vi "Convert Dirs to VI Libraries (proxy)__ogtk.vi"(8 "error in (no error)":errorcluster, 11 "directories":path[](array[path])) -> (0 "error out":errorcluster)   [LabVIEW 2011]
doc: "Converts an array of Directories into VI Library (.llb) files. \n\nNote: This VI dynamically calls the LabVIEW subVI \"Convert Dirs to VI Libraries.vi\" located at <LabVIEW>\\project\\llbedit.llb (as it is not in the VI search paths)."
uses:
  Convert File Extension (Path)__ogtk.vi
panel:
  in  "type specifier":refnum<vi>
  # "Convert Dirs to VI Libraries (proxy).vi\n\nCalls \"Convert Dirs to VI Libraries.vi\" by reference\n\nPlease visit http://www.OpenG.org to learn about the\nOpen Source LabVIEW software movement.\n\nNOTICE -- YOU MUST LEAVE THIS NOTICE IN PLACE.  PER THE TERMS OF THE LICENSE BELOW, YOU MAY SUBLICENSE THIS SOFTWARE \nIN ANY WAY THAT DOES NOT CONFLICT WITH THIS LICENSE.\n\n### BSD License (http://www.opensource.org/licenses/bsd-license.php) Begin ###\n \nCopyright (c) 2003-2006, Jim Kring <jim@jimkring.com>\n\nAll rights reserved.\n\nRedistribution and use in source and binary forms, with or without modification, are permitted provided that the following conditions are met:\n\n    * Redistributions of source code must retain the above copyright notice, this list of conditions and the following disclaimer.\n    * Redistributions in binary form must reproduce the above copyright notice, this list of conditions and the following disclaimer in the \n       documentation and/or other materials provided with the distribution.\n    * Neither the name of SciWare, James Kring, Inc., nor the names of its contributors may be used to endorse or promote products derived \n       from this software without specific prior written permission.\n\nTHIS SOFTWARE IS PROVIDED BY THE COPYRIGHT HOLDERS AND CONTRIBUTORS \"AS IS\" AND ANY EXPRESS OR IMPLIED WARRANTIES, \nINCLUDING, BUT NOT LIMITED TO, THE IMPLIED WARRANTIES OF MERCHANTABILITY AND FITNESS FOR A PARTICULAR PURPOSE ARE \nDISCLAIMED. IN NO EVENT SHALL THE COPYRIGHT OWNER OR CONTRIBUTORS BE LIABLE FOR ANY DIRECT, INDIRECT, INCIDENTAL,\n SPECIAL, EXEMPLARY, OR CONSEQUENTIAL DAMAGES (INCLUDING, BUT NOT LIMITED TO, PROCUREMENT OF SUBSTITUTE GOODS OR \nSERVICES; LOSS OF USE, DATA, OR PROFITS; OR BUSINESS INTERRUPTION) HOWEVER CAUSED AND ON ANY THEORY OF LIABILITY, \nWHETHER IN CONTRACT, STRICT LIABILITY, OR TORT (INCLUDING NEGLIGENCE OR OTHERWISE) ARISING IN ANY WAY OUT OF THE USE \nOF THIS SOFTWARE, EVEN IF ADVISED OF THE POSSIBILITY OF SUCH DAMAGE.\n\n### BSD License End ###"
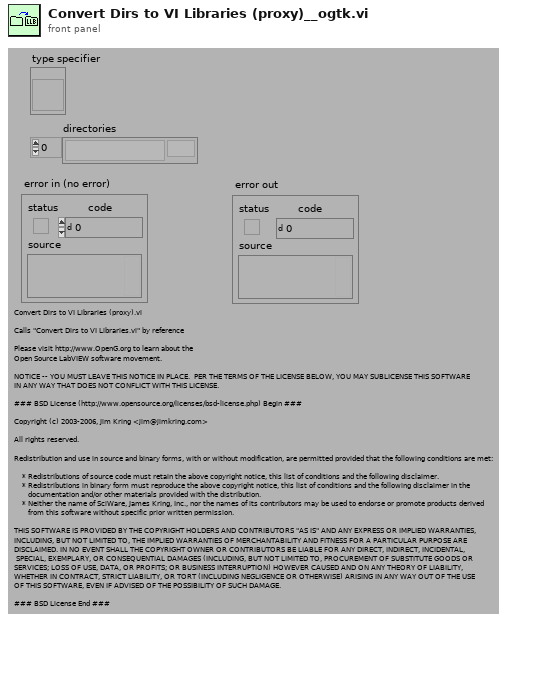
[diagram p1: front panel]
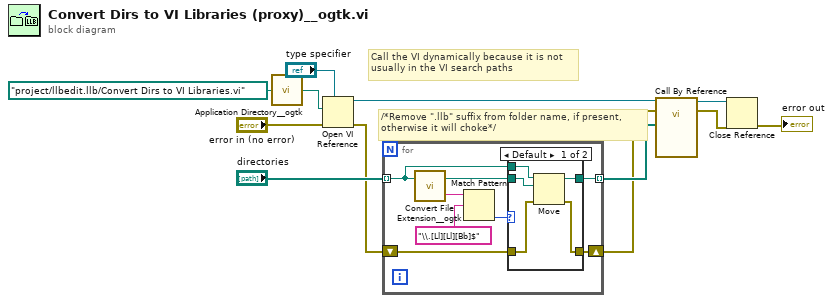
[diagram p0: block diagram]
diagram:
  # "/*Remove \".llb\" suffix from folder name, if present,\notherwise it will choke*/"
  # "Call the VI dynamically because it is not\nusually in the VI search paths"
  n1 = call "Application Directory__ogtk.vi"("Relative path (.)"=path "project/llbedit.llb/Convert Dirs to VI Libraries.vi") -> ("Application Directory (+ Relative)"=w5:path)
  n2 = Open VI Reference(type specifier VI Refnum (for type only)="type specifier", vi path=w5, error in (no error)="error in (no error)") -> (vi reference=w11:refnum<vi>, error out=w1:errorcluster)  [unwired: 3 in]
  n3 = for {
    tunnel: "directories" -> [w16] mode=indexing
    tunnel: [w15] -> w3 mode=indexing
    shift-right: [w13] -> w2
    shift-left: w1 -> [w14]
    n4 = call-poly "Convert File Extension__ogtk.vi"("file name"=w16) -> ("prev ending"=w20:string, "new filename"=w17:path)  [unwired: 1 in]
    n5 = Match Pattern(string=w20, regular expression="\\.[Ll][Ll][Bb]$" ("prev ending")) -> (offset past match=w18:i32)  [unwired: 1 in, 3 out]
    n6 = case shown="Default" w18 {
      tunnel: w17 -> [w25 _]
      tunnel: [w23 w27] -> w15
      tunnel: w16 -> [w24 w27]
      tunnel: w14 -> [w22 w26]
      tunnel: [w21 w26] -> w13
      frame Default {
        n7 = Move(source path=w24, error in=w22, 10:w25) -> (error out=w21:errorcluster, 3:w23:path)  [unwired: 2 in, 1 out]
      }
      frame -1 {
      }
    }
  }
  n8 = call-by-ref "?"(reference=w11, error in=w2, "directories"=w3) -> (reference out=w10:refnum<vi>, error out=w9:errorcluster)  [unwired: 11 in]
  n9 = Close Reference(reference=w10, error in (no error)=w9) -> (error out=→"error out":errorcluster)
